vi "Write connection type.vi"(8 "error in (no error)":errorcluster, 10 "connection type":T1, 11 "tcp connection in":refnum<class "tcp connection.lvclass">) -> (0 "error out":errorcluster, 3 "tcp connection out":refnum<class "tcp connection.lvclass">)   [LabVIEW 2014, in "tcp connection.lvclass"]
uses:
  tcp connection.lvclass
  typedefs/connection type.ctl
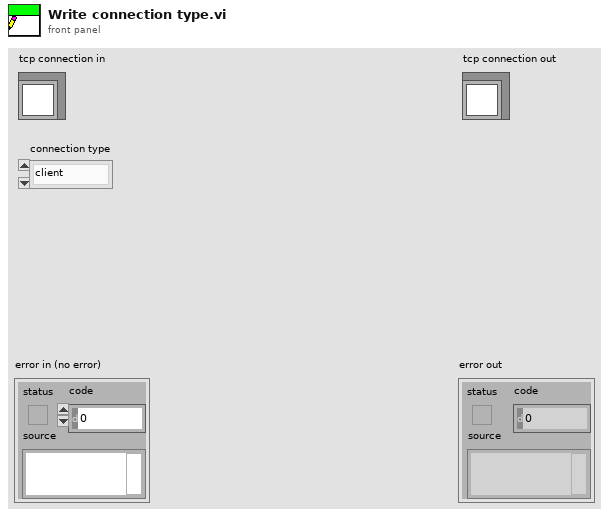
[diagram p1: front panel]
types:
  T1 = typedef "connection type.ctl" = enum16{"client", "server"}
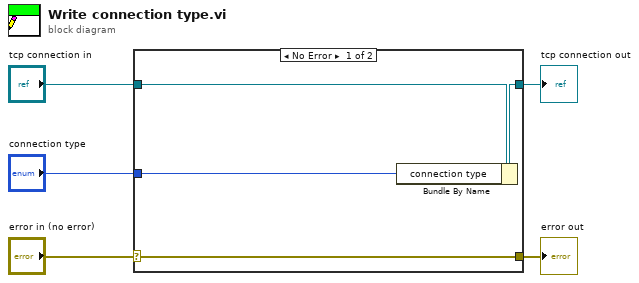
[diagram p0: block diagram]
diagram:
  n1 = case shown="No Error" "error in (no error)" {
    selector: "error in (no error)" -> [w9 w10]
    tunnel: [w9 w10] -> w4
    tunnel: [w7 w11] -> w2
    tunnel: "tcp connection in" -> [w8 w11]
    tunnel: "connection type" -> [w6 _]
    frame No Error {
      n2 = Bundle By Name(cluster=w8, "connection type"=w6) -> (w7:refnum<class "tcp connection.lvclass">)
    }
    frame Error {
    }
  }
  "error out" <- w4
  "tcp connection out" <- w2
